vi "Enable.vi"(8 "error in (no error)":errorcluster, 10 "Enable":bool, 11 "Spring Motor in":refnum<class "Spring Motor.lvclass">) -> (0 "error out":errorcluster, 2 "Message":string, 3 "Spring Motor out":refnum<class "Spring Motor.lvclass">)   [LabVIEW 2021, in "Spring Motor.lvclass"]
uses:
  Spring Motor.lvclass
  Actuator/Actuator.lvclass
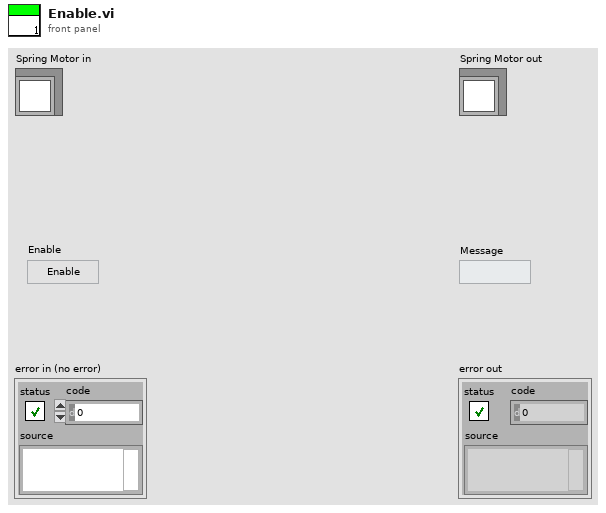
[diagram p1: front panel]
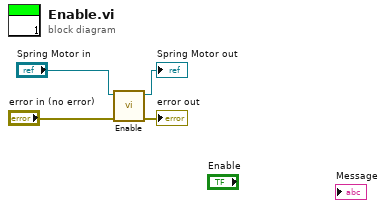
[diagram p0: block diagram]
diagram:
  n1 = call-parent "Enable.vi"("error in (no error)"="error in (no error)", "Actuator in"="Spring Motor in") -> ("error out"=→"error out":errorcluster, "Actuator out"=→"Spring Motor out":refnum<class "Spring Motor.lvclass">)  [unwired: 7 in, 1 out]
